vi "Start STD Cal Data.vi"(8 "에러 입력":errorcluster caption="에러 입력(에러 없음)", 11 "Func_ext":string) -> (0 "에러 출력":errorcluster, 1 "Func_ext Out":string, 2 "기준기명 out":string[](array[string]), 3 "Cal STD":string[][](array[string]), 4 "Func_ext_R제거":string, 5 "Condition":string[][](array[string]), 6 "세부분류코드":string, 7 "Condition Default":string[][](array[string]))   [LabVIEW 2020]
uses:
  Controls/Cmd_Var Data IO.ctl
  Variables/Global_Cal STD.vi
  Public/Polymorph/Array Dedup_1D Str.vi
  Variables/Global_Cal Info.vi
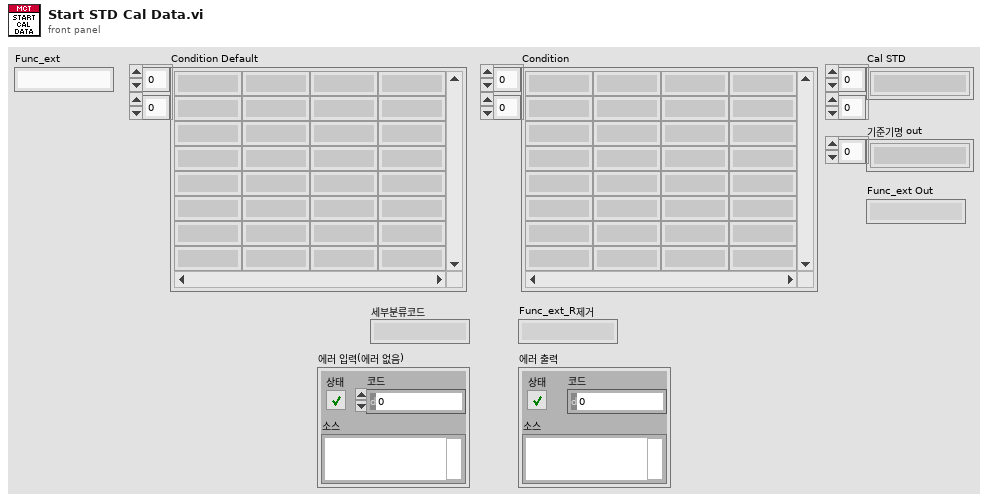
[diagram p1: front panel]
types:
  T1 = typedef "Cmd_Var Data IO.ctl" = enum16{"Condition", "Condition Default", "Condition_Temp", "Resolution", "Resolution Default", "Resolution Old", "Spec", "Spec Default", "Spec Old", "Spec Temp", "Result", "Result2", "Result3", "Result_Temp", "Result_ADJ", "Result_ADJ2", "STD1", "STD2", "STD3", "STD4", "STD5", "STD Temp", "CMC", "CMC Default"}
  T2 = cluster{"세부분류코드":string, "형식":string, "옵션":string, "측정기명":string, "EXCEL파일명":string, "TEMP":string}
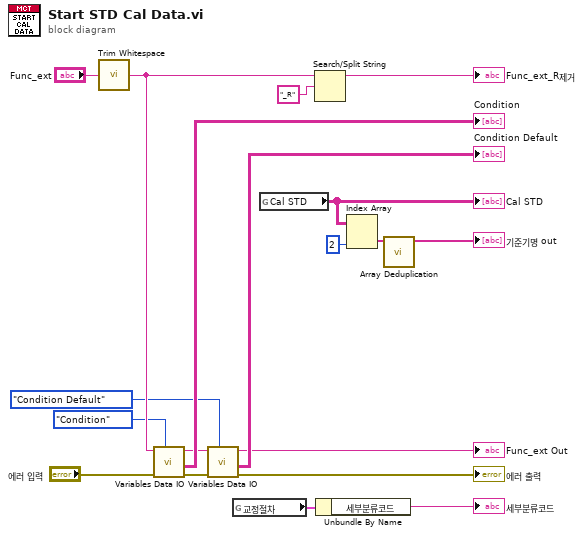
[diagram p0: block diagram]
diagram:
  n1 = call <vilib>:"Trim Whitespace.vi"("string"="Func_ext") -> ("trimmed string"=w12:string)  [unwired: 1 in]
  n2 = call "Variables Data IO.vi"("Select"=Cmd_Var_Data_IO."Condition", "error in"="에러 입력", "Func_ext"=w12) -> ("error out"=w5:errorcluster, "Data Out"=→"Condition":string[][], "Func_ext Out"=w7:string)  [unwired: 6 in]
  n3 = call "Variables Data IO.vi"("Select"=Cmd_Var_Data_IO."Condition Default", "error in"=w5, "Func_ext"=w7) -> ("error out"=→"에러 출력":errorcluster, "Data Out"=→"Condition Default":string[][], "Func_ext Out"=→"Func_ext Out":string)  [unwired: 6 in]
  n4 = global read "Global_Cal Info.vi" "교정절차"() -> (w15:T2)
  n5 = global read "Global_Cal STD.vi" "Cal STD"() -> (w1:string[][])
  "Cal STD" <- w1
  n6 = Search/Split String(string=w12, search string/char (-)="_R" ("검색 문자열/문자 (-)")) -> (substring before match=→"Func_ext_R제거":string)  [unwired: 1 in, 2 out]
  n7 = Unbundle By Name(w15) -> ("세부분류코드"=→"세부분류코드":string)
  n8 = Index Array(array=w1, index (col)=2 ("비활성화된 인덱스 (열)")) -> (element=w17:string[])  [unwired: 1 in]
  n9 = call-poly "Array Deduplication.vi"("배열 in"=w17) -> ("배열 out"=→"기준기명 out":string[])  [unwired: 9 in, 1 out]
